vi "read_raw_record.vi"(8 "error in":errorcluster, 11 "Byte Stream File in":refnum<file>) -> (0 "error out":errorcluster, 1 "Input data":waveform(dbl)[][](array[waveform]), 2 "Timestamps":timestamp[](array[timestamp]), 3 "Byte Stream File out":refnum<file>)   [LabVIEW 2014]
uses:
  main/ilemt_globals.vi
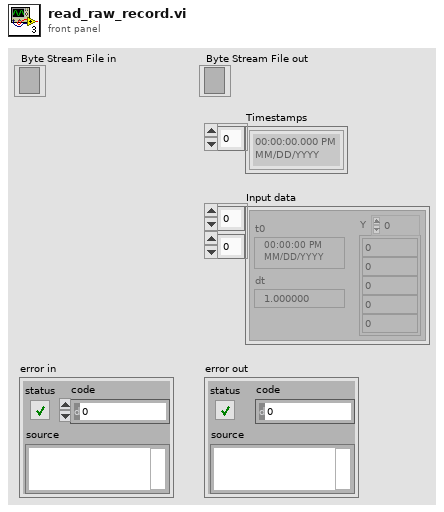
[diagram p1: front panel]
types:
  T1 = typedef "modulation_info.ctl" = cluster{"Fs full":dbl, "Fs high":dbl, "Fs low":dbl, "Read size":i32, "FFT size low":i32, "df low":dbl, "High carriers":dbl[], "Low carriers":dbl[], "Hi channels at low":i32[]}
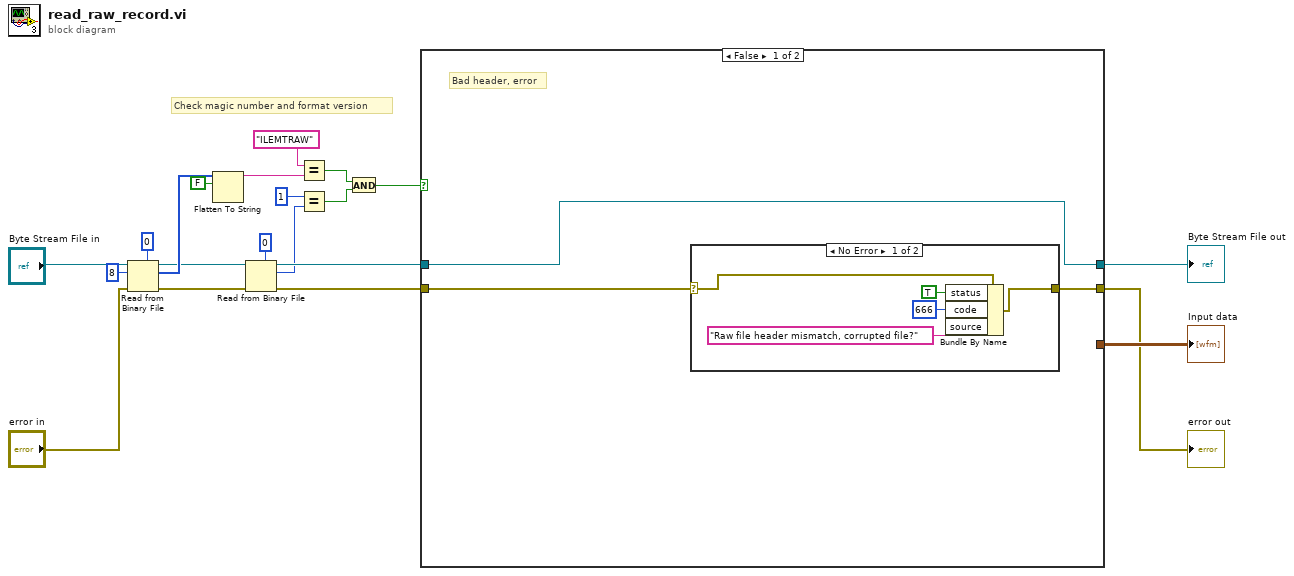
[diagram p0: block diagram]
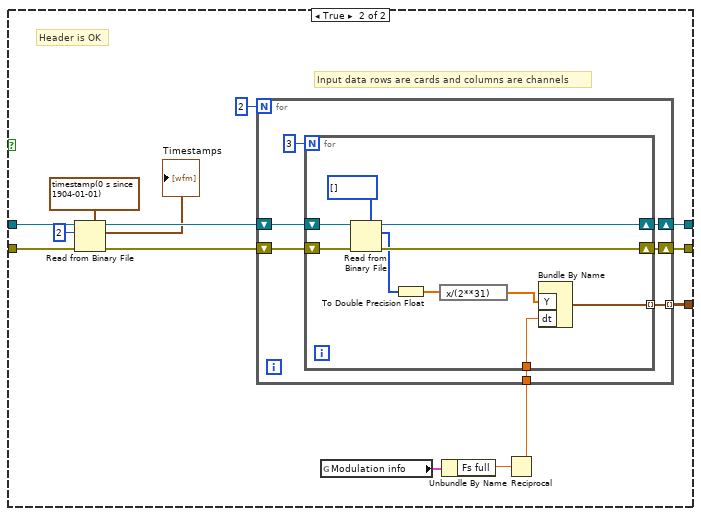
[diagram p3: hidden frame]
diagram:
  # "Check magic number and format version"
  n1 = Read from Binary File(5:u8 0, 8:"error in", 10:8 ("count (1)"), 11:"Byte Stream File in") -> (0:w15:errorcluster, 2:w19:u8[], 3:w12:refnum<file>)  [unwired: 2 in, 1 out]
  n2 = Flatten To String(anything=w19, prepend array or string size? (T)=FALSE) -> (data string=w7:string)  [unwired: 2 in, 2 out]
  n3 = Read from Binary File(5:0, 8:w15, 11:w12) -> (0:w16:errorcluster, 2:w5:i32, 3:w13:refnum<file>)  [unwired: 3 in, 1 out]
  n4 = Equal?(x="ILEMTRAW", y=w7) -> (x = y?=w3:bool)
  n5 = Equal?(x=1, y=w5) -> (x = y?=w2:bool)
  n6 = And(x=w3, y=w2) -> (x .and. y?=w1:bool)
  n7 = case shown="False" w1 {
    tunnel: [_ w44] -> w21
    tunnel: [w23 w39] -> w18
    tunnel: [w24 w38] -> w17
    tunnel: w16 -> [w22 w33]
    tunnel: w13 -> [w24 w32]
    frame False {
      # "Bad header, error"
      n8 = case shown="No Error" w22 {
        selector: w22 -> [w25 w30]
        tunnel: [w29 w30] -> w23
        frame No Error {
          n9 = Bundle By Name(cluster=w25, "status"=TRUE, "code"=666, "source"="Raw file header mismatch, corrupted file?") -> (w29:errorcluster)
        }
        frame Error {
        }
      }
    }
    frame True {
      # "Header is OK"
      # "Input data rows are cards and columns are channels"
      n10 = Read from Binary File(5:timestamp(0 s since 1904-01-01) ("current time"), 8:w33, 10:2 ("count (1)"), 11:w32) -> (0:w37:errorcluster, 2:→"Timestamps":timestamp[], 3:w36:refnum<file>)  [unwired: 2 in, 1 out]
      n11 = global read "ilemt_globals.vi" "Modulation info"() -> (w40:T1)
      n12 = Unbundle By Name(w40) -> ("Fs full"=w41:dbl)
      n13 = Reciprocal(x=w41) -> (1/x=w42:dbl)
      n14 = for {
        N: 2 -> [_]
        tunnel: w42 -> [w47]
        shift-right: [w49] -> w38
        shift-left: w36 -> [w51]
        shift-right: [w48] -> w39
        shift-left: w37 -> [w50]
        tunnel: [w45] -> w44 mode=indexing
        n15 = for {
          N: 3 -> [_]
          tunnel: w47 -> [w53]
          shift-right: [w58] -> w49
          shift-left: w51 -> [w60]
          shift-right: [w57] -> w48
          shift-left: w50 -> [w59]
          tunnel: [w52] -> w45 mode=indexing
          n16 = Read from Binary File(5:i32[] [] ("32bit integer"), 8:w59, 11:w60) -> (0:w57:errorcluster, 2:w56:i32[], 3:w58:refnum<file>)  [unwired: 3 in, 1 out]
          n17 = To Double Precision Float(number=w56) -> (double precision float=w55:dbl[])
          n18 = expression code="x/(2**31)"(w55) -> (w54:dbl[])
          n19 = Bundle By Name("Y"=w54, "dt"=w53) -> (w52:waveform(dbl))  [unwired: 1 in]
        }
      }
    }
  }
  "Input data" <- w21
  "error out" <- w18
  "Byte Stream File out" <- w17
